vi "file -- coerse folder and file.vi"(9 "sweep folder":path, 11 "file":path) -> (3 "sweep file":path)   [LabVIEW 2015]
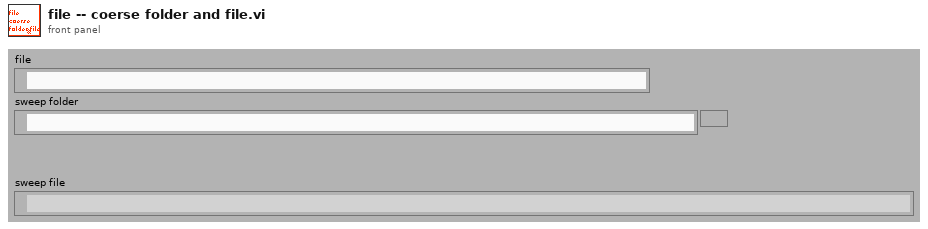
[diagram p1: front panel]
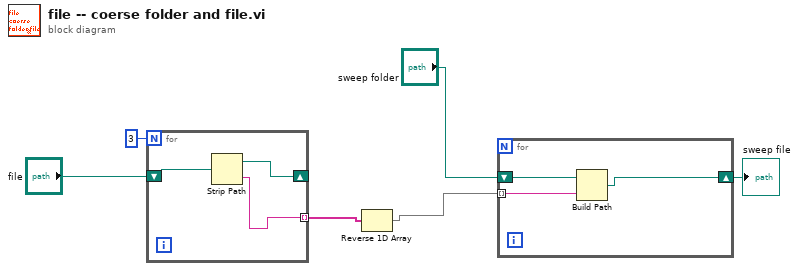
[diagram p0: block diagram]
diagram:
  n1 = for {
    N: 3 -> [_]
    shift-right: [w8] -> _
    shift-left: "file" -> [w9]
    tunnel: [w7] -> w4 mode=indexing
    n2 = Strip Path(path=w9) -> (stripped path=w8:path, name=w7:string)
  }
  n3 = Reverse 1D Array(array=w4) -> (reversed array=w2:string[])
  n4 = for {
    tunnel: w2 -> [w11] mode=indexing
    shift-right: [w10] -> w1
    shift-left: "sweep folder" -> [w12]
    n5 = Build Path(base path=w12, name or relative path=w11) -> (appended path=w10:path)
  }
  "sweep file" <- w1
